vi "TIO SLIP Serial Read.vi"(8 "error in (no error)":errorcluster, 11 "VISA resource name":refnum<visa-resource-name>) -> (0 "error out":errorcluster, 1 "CRC32":bool, 2 "Payload":string, 3 "VISA resource name Out":refnum<visa-resource-name>)   [LabVIEW 2019]
panel:
  out "Raw buffer":string
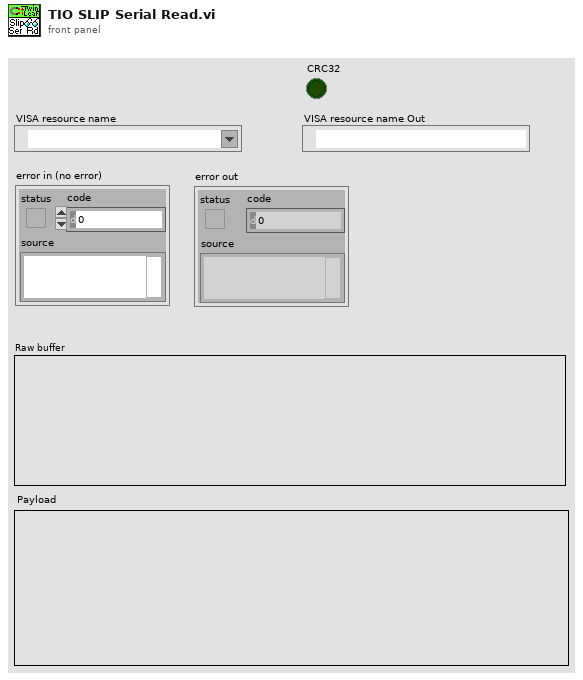
[diagram p1: front panel]
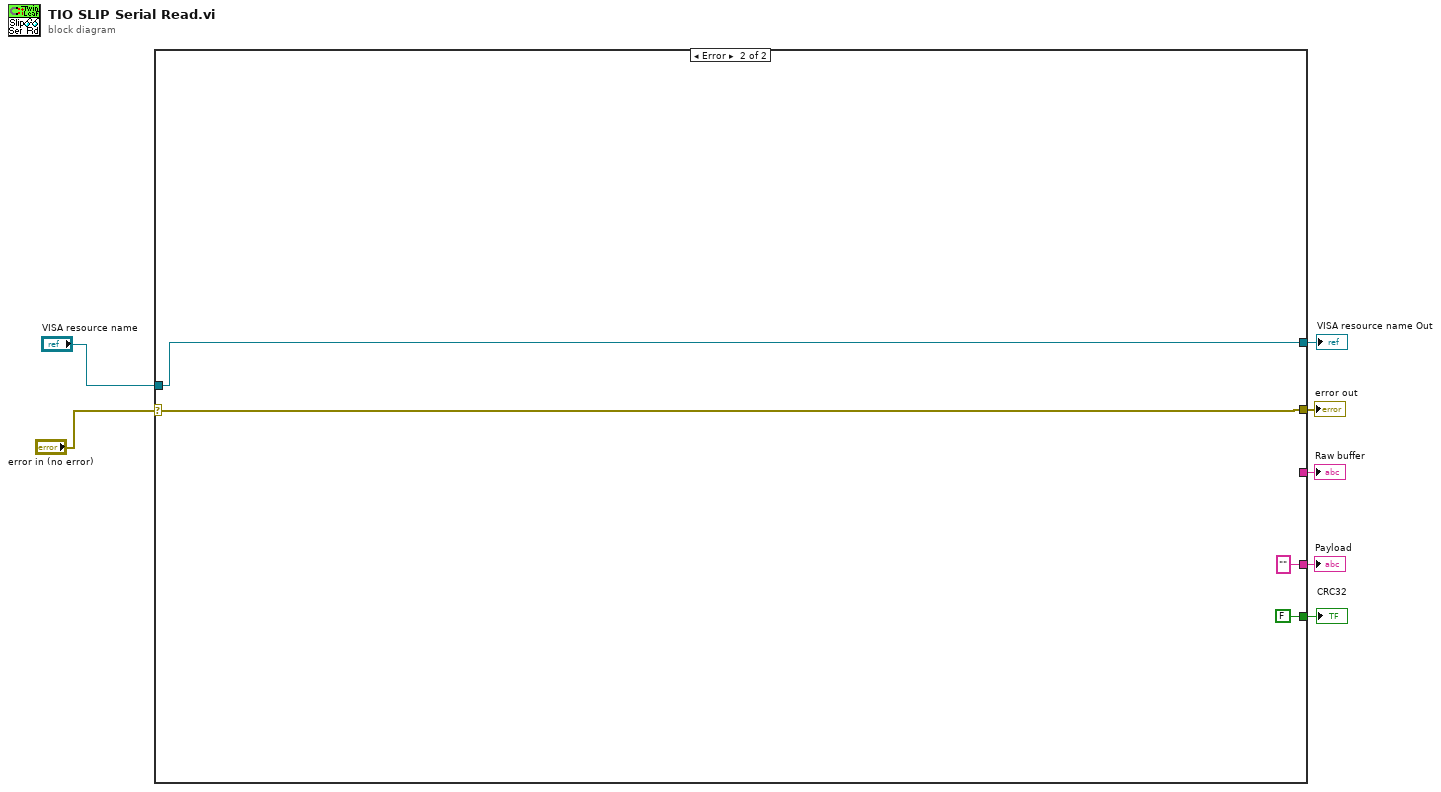
[diagram p0: block diagram]
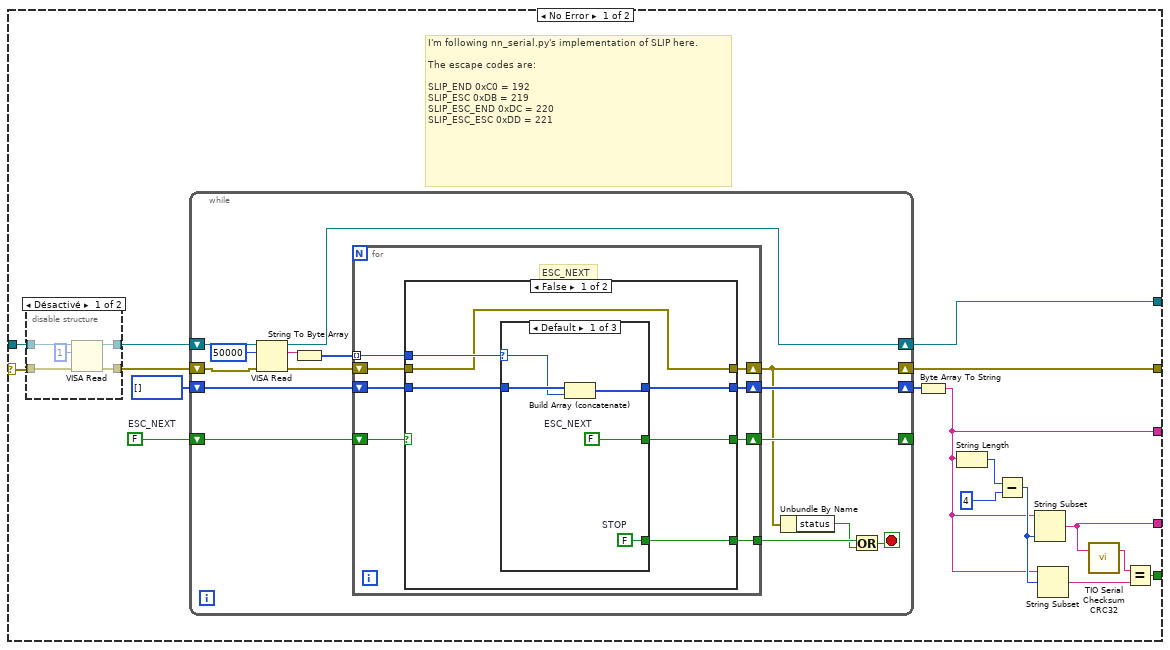
[diagram p2: hidden frame]
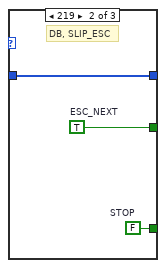
[diagram p4: hidden frame]
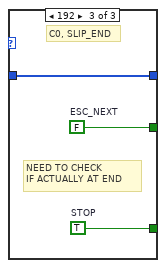
[diagram p5: hidden frame]
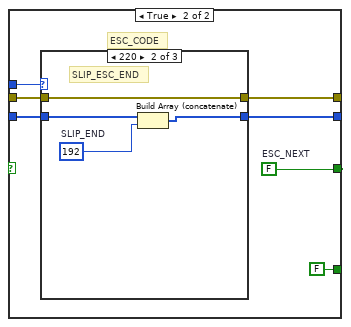
[diagram p6: hidden frame]
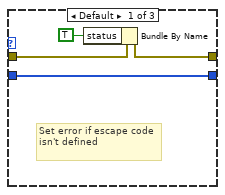
[diagram p7: hidden frame]
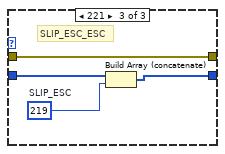
[diagram p8: hidden frame]
diagram:
  n1 = case shown="Error" "error in (no error)" {
    selector: "error in (no error)" -> [w8 w94]
    tunnel: [w24 w93] -> w7
    tunnel: [w23 w94] -> w6
    tunnel: "VISA resource name" -> [w19 w93]
    tunnel: [w13 "" ("string")] -> w4
    tunnel: [w11 FALSE] -> w3
    tunnel: [w10 _] -> w2
    frame No Error {
      w21 = FALSE  # ESC_NEXT
      # "I'm following nn_serial.py's implementation of SLIP here. \n\nThe escape codes are:\n\nSLIP_END\t0xC0 = 192\nSLIP_ESC\t0xDB = 219\nSLIP_ESC_END\t0xDC = 220\nSLIP_ESC_ESC\t0xDD = 221"
      n2 = disable-structure shown="Désactivé" {
        disable-tunnel: w19 -> [w29 w31]
        disable-tunnel: [w28 w31] -> w18
        disable-tunnel: [w27 w30] -> w17
        disable-tunnel: w8 -> [w26 w30]
        frame Disabled {
          n3 = VISA Read(VISA resource name=w29, byte count=u32 1, error in (no error)=w26) -> (VISA resource name out=w28:refnum<visa-resource-name>, error out=w27:errorcluster)  [unwired: 2 out]
        }
        frame Enabled {
        }
      }
      n4 = while {
        shift-right: [w40] -> w20
        shift-left: u8[] [] ("unsigned byte array") -> [w46]
        shift-right: [w32] -> w24
        shift-left: w18 -> [w34]
        shift-right: [w37] -> w23
        shift-left: w17 -> [w33]
        shift-right: [w43] -> _
        shift-left: w21 -> [w45]
        stop <- w38 stop-if-true
        n5 = VISA Read(VISA resource name=w34, byte count=u32 50000, error in (no error)=w33) -> (VISA resource name out=w32:refnum<visa-resource-name>, read buffer=w44:string, error out=w42:errorcluster)  [unwired: 1 out]
        n6 = String To Byte Array(string=w44) -> (unsigned byte array=w41:u8[])
        n7 = for {
          tunnel: [w51] -> w39
          shift-right: [w52] -> w43
          shift-left: w45 -> [w53]
          shift-right: [w49] -> w37
          shift-left: w42 -> [w50]
          tunnel: w41 -> [w48] mode=indexing
          shift-right: [w47] -> w40
          shift-left: w46 -> [w54]
          # "ESC_NEXT"
          n8 = case shown="False" w53 {
            tunnel: w54 -> [w60 w78]
            tunnel: [w59 w77] -> w47
            tunnel: w48 -> [w57 w76]
            tunnel: [w58 w75] -> w52
            tunnel: [w55 w74] -> w49
            tunnel: [w56 FALSE ("STOP")] -> w51
            tunnel: w50 -> [w55 w72]
            frame False {
              n9 = case shown="Default" w57 {
                selector: w57 -> [w64 _ _]
                tunnel: w60 -> [w65 w68 w71]
                tunnel: [w63 w68 w71] -> w59
                tunnel: [w62 w67 w70] -> w58
                tunnel: [w61 w66 w69] -> w56
                frame Default {
                  w61 = FALSE  # STOP
                  w62 = FALSE  # ESC_NEXT
                  n10 = Build Array (concatenate)(w65, w64) -> (w63:u8[])
                }
                frame 219 {
                  w66 = FALSE  # STOP
                  w67 = TRUE  # ESC_NEXT
                  # "DB, SLIP_ESC"
                }
                frame 192 {
                  w69 = TRUE  # STOP
                  w70 = FALSE  # ESC_NEXT
                  # "NEED TO CHECK\nIF ACTUALLY AT END"
                  # "C0, SLIP_END"
                }
              }
            }
            frame True {
              w75 = FALSE  # ESC_NEXT
              # "ESC_CODE"
              n11 = case shown="220" w76 {
                tunnel: w78 -> [w80 w85 w89]
                tunnel: [w80 w84 w88] -> w77
                tunnel: [w82 w83 w87] -> w74
                tunnel: w72 -> [w79 w83 w87]
                frame Default {
                  # "Set error if escape code isn't defined"
                  n12 = Bundle By Name(cluster=w79, "status"=TRUE) -> (w82:errorcluster)
                }
                frame 220 {
                  w86 = u8 192  # SLIP_END
                  # "SLIP_ESC_END"
                  n13 = Build Array (concatenate)(w85, w86) -> (w84:u8[])
                }
                frame 221 {
                  w90 = u8 219  # SLIP_ESC
                  # "SLIP_ESC_ESC"
                  n14 = Build Array (concatenate)(w89, w90) -> (w88:u8[])
                }
              }
            }
          }
        }
        n15 = Unbundle By Name(w37) -> ("status"=w36:bool)
        n16 = Or(x=w39, y=w36) -> (x .or. y?=w38:bool)
      }
      n17 = Byte Array To String(unsigned byte array=w20) -> (string=w10:string)
      n18 = String Length(string=w10) -> (length=w16:i32)
      n19 = Subtract(x=w16, y=4) -> (x-y=w14:i32)
      n20 = String Subset(string=w10, length (rest)=w14) -> (substring=w13:string)  [unwired: 1 in]
      n21 = String Subset(string=w10, offset (0)=w14) -> (substring=w9:string)  [unwired: 1 in]
      n22 = call <userlib>:"TIO Serial Checksum CRC32.vi"("String"=w13) -> ("CRC32 Little Endian String"=w12:string)  [unwired: 1 in, 1 out]
      n23 = Equal?(x=w12, y=w9) -> (x = y?=w11:bool)
    }
    frame Error {
    }
  }
  "error out" <- w6
  "Payload" <- w4
  "VISA resource name Out" <- w7
  "CRC32" <- w3
  "Raw buffer" <- w2
